vi "F2Value.vi"(3 "channel 2":dbl[](array[numeric]) format="%.2f", 4 "channel1":dbl[](array[numeric]) format="%.2f", 5 "Index Hi":u32[](array[numeric]), 6 "Index Low":u32[](array[numeric])) -> (0 "channel2 out":dbl[](array[numeric]) format="%.2f", 1 "channel1 out":dbl[](array[numeric]) format="%.2f", 2 "F2-values":dbl[](array[numeric]) format="%.2f")   [LabVIEW 2009]
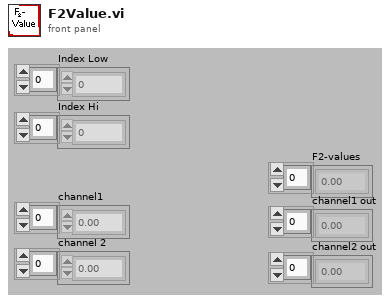
[diagram p1: front panel]
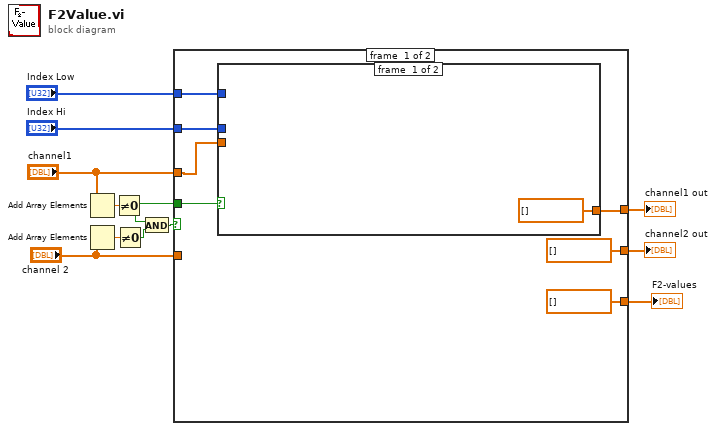
[diagram p0: block diagram]
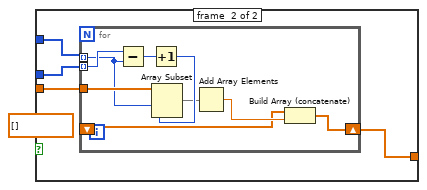
[diagram p2: hidden frame]
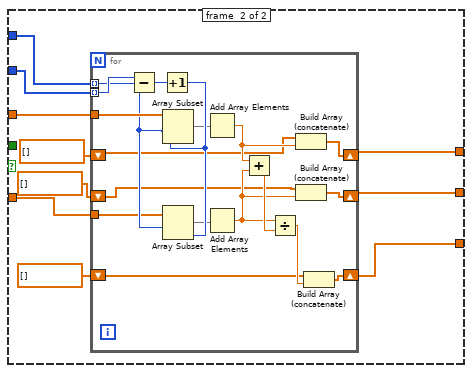
[diagram p3: hidden frame]
diagram:
  n1 = Add Array Elements(numeric array="channel1") -> (sum=w9:dbl)
  n2 = Add Array Elements(numeric array="channel 2") -> (sum=w8:dbl)
  n3 = Not Equal To 0?(x=w9) -> (x != 0?=w1:bool)
  n4 = Not Equal To 0?(x=w8) -> (x != 0?=w6:bool)
  n5 = And(x=w1, y=w6) -> (x .and. y?=w5:bool)
  n6 = case shown="True" w5 {
    tunnel: "Index Hi" -> [w15 w42]
    tunnel: "Index Low" -> [w16 w41]
    tunnel: "channel 2" -> [_ w40]
    tunnel: "channel1" -> [w14 w39]
    tunnel: [w13 w36] -> w4
    tunnel: [dbl[] [] w35] -> w3
    tunnel: [dbl[] [] w34] -> w2
    tunnel: w1 -> [w17 _]
    frame #0 {
      n7 = case shown="True" w17 {
        tunnel: w16 -> [_ w24]
        tunnel: w15 -> [_ w23]
        tunnel: w14 -> [_ w22]
        tunnel: [dbl[] [] w21] -> w13
        frame #0 {
        }
        frame #1 {
          (unwired) dbl[] []
          n8 = for {
            tunnel: w22 -> [w32]
            tunnel: w24 -> [w30] mode=indexing
            tunnel: w23 -> [w33] mode=indexing
            shift-right: [w26] -> w21
            shift-left: _ -> [w25]
            n9 = Subtract(x=w33, y=w30) -> (x-y=w31:u32)
            n10 = Increment(x=w31) -> (x+1=w29:u32)
            n11 = Array Subset(array=w32, index=w30, length=w29) -> (w28:dbl[])
            n12 = Add Array Elements(numeric array=w28) -> (sum=w27:dbl)
            n13 = Build Array (concatenate)(w25, w27) -> (w26:dbl[])
          }
        }
      }
    }
    frame #1 {
      n14 = for {
        tunnel: w39 -> [w60]
        tunnel: w40 -> [w56]
        tunnel: w41 -> [w58] mode=indexing
        tunnel: w42 -> [w61] mode=indexing
        shift-right: [w51] -> w34
        shift-left: dbl[] [] -> [w50]
        shift-right: [w46] -> w35
        shift-left: dbl[] [] -> [w44]
        shift-right: [w48] -> w36
        shift-left: dbl[] [] -> [w45]
        n15 = Subtract(x=w61, y=w58) -> (x-y=w59:u32)
        n16 = Increment(x=w59) -> (x+1=w57:u32)
        n17 = Array Subset(array=w60, index=w58, length=w57) -> (w54:dbl[])
        n18 = Array Subset(array=w56, index=w58, length=w57) -> (w55:dbl[])
        n19 = Add Array Elements(numeric array=w54) -> (sum=w49:dbl)
        n20 = Add Array Elements(numeric array=w55) -> (sum=w47:dbl)
        n21 = Add(x=w49, y=w47) -> (x+y=w53:dbl)
        n22 = Divide(x=w47, y=w53) -> (x/y=w52:dbl)
        n23 = Build Array (concatenate)(w45, w49) -> (w48:dbl[])
        n24 = Build Array (concatenate)(w44, w47) -> (w46:dbl[])
        n25 = Build Array (concatenate)(w50, w52) -> (w51:dbl[])
      }
    }
  }
  "channel1 out" <- w4
  "channel2 out" <- w3
  "F2-values" <- w2
